vi "校准数据写入配置文件.vi"(8 "error in (no error)":errorcluster) -> (0 "error out":errorcluster)   [LabVIEW 2016, in "斯坦道通用流路CODmn.lvlib"]
uses:
  <vilib>/Utility/config.llb/NI_LVConfig.lvlib
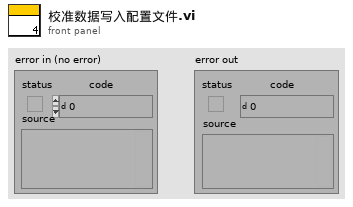
[diagram p1: front panel]
types:
  T1 = cluster{"参数":cluster{"String":string, "Value":u16}, "曲线模型":cluster{"标液浓度1":dbl, "测量吸光度1":dbl, "样品1启用":bool, "标液浓度2":dbl, "测量吸光度2":dbl, "样品2启用":bool, "标液浓度3":dbl, "测量吸光度3":dbl, "样品3启用":bool, "标液浓度4":dbl, "测量吸光度4":dbl, "样品4启用":bool, "标液浓度5":dbl, "测量吸光度5":dbl, "样品5启用":bool, "模型":enum32{"线性", "多项式"}, "精度":dbl, "XY图":cluster{"X Values":dbl[], "Y Values":dbl[]}[], "拟合公式":string, "r^2":dbl, "标样一校准时间":timestamp, "标样二校准时间":timestamp, "标样三校准时间":timestamp, "标样四校准时间":timestamp, "标样五校准时间":timestamp, "方程":cluster{"c":dbl, "x":dbl, "x^2":dbl}, "标定时间":timestamp}[]}[]
  T2 = cluster{"标液浓度1":dbl, "测量吸光度1":dbl, "样品1启用":bool, "标液浓度2":dbl, "测量吸光度2":dbl, "样品2启用":bool, "标液浓度3":dbl, "测量吸光度3":dbl, "样品3启用":bool, "标液浓度4":dbl, "测量吸光度4":dbl, "样品4启用":bool, "标液浓度5":dbl, "测量吸光度5":dbl, "样品5启用":bool, "模型":enum32{"线性", "多项式"}, "精度":dbl, "XY图":cluster{"X Values":dbl[], "Y Values":dbl[]}[], "拟合公式":string, "r^2":dbl, "标样一校准时间":timestamp, "标样二校准时间":timestamp, "标样三校准时间":timestamp, "标样四校准时间":timestamp, "标样五校准时间":timestamp, "二次方程":cluster{"c":dbl, "x":dbl, "x^2":dbl}, "标定时间":timestamp}[]
  T3 = cluster{cluster{"String":string, "Value":u16}, "总磷曲线模型":cluster{"标液浓度1":dbl, "测量吸光度1":dbl, "样品1启用":bool, "标液浓度2":dbl, "测量吸光度2":dbl, "样品2启用":bool, "标液浓度3":dbl, "测量吸光度3":dbl, "样品3启用":bool, "标液浓度4":dbl, "测量吸光度4":dbl, "样品4启用":bool, "标液浓度5":dbl, "测量吸光度5":dbl, "样品5启用":bool, "模型":enum32{"线性", "多项式"}, "精度":dbl, "XY图":cluster{"X Values":dbl[], "Y Values":dbl[]}[], "拟合公式":string, "r^2":dbl, "标样一校准时间":timestamp, "标样二校准时间":timestamp, "标样三校准时间":timestamp, "标样四校准时间":timestamp, "标样五校准时间":timestamp, "二次方程":cluster{"c":dbl, "x":dbl, "x^2":dbl}, "标定时间":timestamp}[]}
  T4 = cluster{cluster{"String":string, "Value":u16}, "总氮曲线模型":cluster{"标液浓度1":dbl, "测量吸光度1":dbl, "样品1启用":bool, "标液浓度2":dbl, "测量吸光度2":dbl, "样品2启用":bool, "标液浓度3":dbl, "测量吸光度3":dbl, "样品3启用":bool, "标液浓度4":dbl, "测量吸光度4":dbl, "样品4启用":bool, "标液浓度5":dbl, "测量吸光度5":dbl, "样品5启用":bool, "模型":enum32{"线性", "多项式"}, "精度":dbl, "XY图":cluster{"X Values":dbl[], "Y Values":dbl[]}[], "拟合公式":string, "r^2":dbl, "标样一校准时间":timestamp, "标样二校准时间":timestamp, "标样三校准时间":timestamp, "标样四校准时间":timestamp, "标样五校准时间":timestamp, "二次方程":cluster{"c":dbl, "x":dbl, "x^2":dbl}, "标定时间":timestamp}[]}
  T5 = cluster{cluster{"String":string, "Value":u16}, "氨氮曲线模型":cluster{"标液浓度1":dbl, "测量吸光度1":dbl, "样品1启用":bool, "标液浓度2":dbl, "测量吸光度2":dbl, "样品2启用":bool, "标液浓度3":dbl, "测量吸光度3":dbl, "样品3启用":bool, "标液浓度4":dbl, "测量吸光度4":dbl, "样品4启用":bool, "标液浓度5":dbl, "测量吸光度5":dbl, "样品5启用":bool, "模型":enum32{"线性", "多项式"}, "精度":dbl, "XY图":cluster{"X Values":dbl[], "Y Values":dbl[]}[], "拟合公式":string, "r^2":dbl, "标样一校准时间":timestamp, "标样二校准时间":timestamp, "标样三校准时间":timestamp, "标样四校准时间":timestamp, "标样五校准时间":timestamp, "二次方程":cluster{"c":dbl, "x":dbl, "x^2":dbl}, "标定时间":timestamp}[]}
  T6 = cluster{cluster{"String":string, "Value":u16}, "磷酸盐曲线模型":cluster{"标液浓度1":dbl, "测量吸光度1":dbl, "样品1启用":bool, "标液浓度2":dbl, "测量吸光度2":dbl, "样品2启用":bool, "标液浓度3":dbl, "测量吸光度3":dbl, "样品3启用":bool, "标液浓度4":dbl, "测量吸光度4":dbl, "样品4启用":bool, "标液浓度5":dbl, "测量吸光度5":dbl, "样品5启用":bool, "模型":enum32{"线性", "多项式"}, "精度":dbl, "XY图":cluster{"X Values":dbl[], "Y Values":dbl[]}[], "拟合公式":string, "r^2":dbl, "标样一校准时间":timestamp, "标样二校准时间":timestamp, "标样三校准时间":timestamp, "标样四校准时间":timestamp, "标样五校准时间":timestamp, "二次方程":cluster{"c":dbl, "x":dbl, "x^2":dbl}, "标定时间":timestamp}[]}
  T7 = cluster{cluster{"String":string, "Value":u16}, "硝氮曲线模型":cluster{"标液浓度1":dbl, "测量吸光度1":dbl, "样品1启用":bool, "标液浓度2":dbl, "测量吸光度2":dbl, "样品2启用":bool, "标液浓度3":dbl, "测量吸光度3":dbl, "样品3启用":bool, "标液浓度4":dbl, "测量吸光度4":dbl, "样品4启用":bool, "标液浓度5":dbl, "测量吸光度5":dbl, "样品5启用":bool, "模型":enum32{"线性", "多项式"}, "精度":dbl, "XY图":cluster{"X Values":dbl[], "Y Values":dbl[]}[], "拟合公式":string, "r^2":dbl, "标样一校准时间":timestamp, "标样二校准时间":timestamp, "标样三校准时间":timestamp, "标样四校准时间":timestamp, "标样五校准时间":timestamp, "二次方程":cluster{"c":dbl, "x":dbl, "x^2":dbl}, "标定时间":timestamp}[]}
  T8 = cluster{cluster{"String":string, "Value":u16}, "亚硝氮曲线模型":cluster{"标液浓度1":dbl, "测量吸光度1":dbl, "样品1启用":bool, "标液浓度2":dbl, "测量吸光度2":dbl, "样品2启用":bool, "标液浓度3":dbl, "测量吸光度3":dbl, "样品3启用":bool, "标液浓度4":dbl, "测量吸光度4":dbl, "样品4启用":bool, "标液浓度5":dbl, "测量吸光度5":dbl, "样品5启用":bool, "模型":enum32{"线性", "多项式"}, "精度":dbl, "XY图":cluster{"X Values":dbl[], "Y Values":dbl[]}[], "拟合公式":string, "r^2":dbl, "标样一校准时间":timestamp, "标样二校准时间":timestamp, "标样三校准时间":timestamp, "标样四校准时间":timestamp, "标样五校准时间":timestamp, "二次方程":cluster{"c":dbl, "x":dbl, "x^2":dbl}, "标定时间":timestamp}[]}
  T9 = cluster{cluster{"String":string, "Value":u16}, "硅酸盐曲线模型":cluster{"标液浓度1":dbl, "测量吸光度1":dbl, "样品1启用":bool, "标液浓度2":dbl, "测量吸光度2":dbl, "样品2启用":bool, "标液浓度3":dbl, "测量吸光度3":dbl, "样品3启用":bool, "标液浓度4":dbl, "测量吸光度4":dbl, "样品4启用":bool, "标液浓度5":dbl, "测量吸光度5":dbl, "样品5启用":bool, "模型":enum32{"线性", "多项式"}, "精度":dbl, "XY图":cluster{"X Values":dbl[], "Y Values":dbl[]}[], "拟合公式":string, "r^2":dbl, "标样一校准时间":timestamp, "标样二校准时间":timestamp, "标样三校准时间":timestamp, "标样四校准时间":timestamp, "标样五校准时间":timestamp, "二次方程":cluster{"c":dbl, "x":dbl, "x^2":dbl}, "标定时间":timestamp}[]}
  T10 = cluster{cluster{"String":string, "Value":u16}, "硫化物曲线模型":cluster{"标液浓度1":dbl, "测量吸光度1":dbl, "样品1启用":bool, "标液浓度2":dbl, "测量吸光度2":dbl, "样品2启用":bool, "标液浓度3":dbl, "测量吸光度3":dbl, "样品3启用":bool, "标液浓度4":dbl, "测量吸光度4":dbl, "样品4启用":bool, "标液浓度5":dbl, "测量吸光度5":dbl, "样品5启用":bool, "模型":enum32{"线性", "多项式"}, "精度":dbl, "XY图":cluster{"X Values":dbl[], "Y Values":dbl[]}[], "拟合公式":string, "r^2":dbl, "标样一校准时间":timestamp, "标样二校准时间":timestamp, "标样三校准时间":timestamp, "标样四校准时间":timestamp, "标样五校准时间":timestamp, "二次方程":cluster{"c":dbl, "x":dbl, "x^2":dbl}, "标定时间":timestamp}[]}
  T11 = cluster{cluster{"String":string, "Value":u16}, "CODcr曲线模型":cluster{"标液浓度1":dbl, "测量吸光度1":dbl, "样品1启用":bool, "标液浓度2":dbl, "测量吸光度2":dbl, "样品2启用":bool, "标液浓度3":dbl, "测量吸光度3":dbl, "样品3启用":bool, "标液浓度4":dbl, "测量吸光度4":dbl, "样品4启用":bool, "标液浓度5":dbl, "测量吸光度5":dbl, "样品5启用":bool, "模型":enum32{"线性", "多项式"}, "精度":dbl, "XY图":cluster{"X Values":dbl[], "Y Values":dbl[]}[], "拟合公式":string, "r^2":dbl, "标样一校准时间":timestamp, "标样二校准时间":timestamp, "标样三校准时间":timestamp, "标样四校准时间":timestamp, "标样五校准时间":timestamp, "二次方程":cluster{"c":dbl, "x":dbl, "x^2":dbl}, "标定时间":timestamp}[]}
  T12 = cluster{cluster{"String":string, "Value":u16}, "CODMn曲线模型":cluster{"标液浓度1":dbl, "测量吸光度1":dbl, "样品1启用":bool, "标液浓度2":dbl, "测量吸光度2":dbl, "样品2启用":bool, "标液浓度3":dbl, "测量吸光度3":dbl, "样品3启用":bool, "标液浓度4":dbl, "测量吸光度4":dbl, "样品4启用":bool, "标液浓度5":dbl, "测量吸光度5":dbl, "样品5启用":bool, "模型":enum32{"线性", "多项式"}, "精度":dbl, "XY图":cluster{"X Values":dbl[], "Y Values":dbl[]}[], "拟合公式":string, "r^2":dbl, "标样一校准时间":timestamp, "标样二校准时间":timestamp, "标样三校准时间":timestamp, "标样四校准时间":timestamp, "标样五校准时间":timestamp, "二次方程":cluster{"c":dbl, "x":dbl, "x^2":dbl}, "标定时间":timestamp}[]}
  T13 = cluster{cluster{"String":string, "Value":u16}, "氟化物曲线模型":cluster{"标液浓度1":dbl, "测量吸光度1":dbl, "样品1启用":bool, "标液浓度2":dbl, "测量吸光度2":dbl, "样品2启用":bool, "标液浓度3":dbl, "测量吸光度3":dbl, "样品3启用":bool, "标液浓度4":dbl, "测量吸光度4":dbl, "样品4启用":bool, "标液浓度5":dbl, "测量吸光度5":dbl, "样品5启用":bool, "模型":enum32{"线性", "多项式"}, "精度":dbl, "XY图":cluster{"X Values":dbl[], "Y Values":dbl[]}[], "拟合公式":string, "r^2":dbl, "标样一校准时间":timestamp, "标样二校准时间":timestamp, "标样三校准时间":timestamp, "标样四校准时间":timestamp, "标样五校准时间":timestamp, "二次方程":cluster{"c":dbl, "x":dbl, "x^2":dbl}, "标定时间":timestamp}[]}
  T14 = typedef "NI_LVConfig.lvlib/Config Data RefNum.ctl" = refnum<k1>
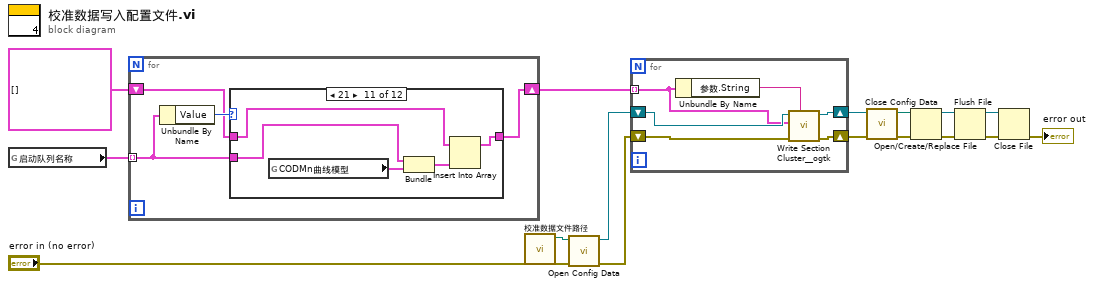
[diagram p0: block diagram]
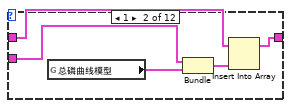
[diagram p3: hidden frame]
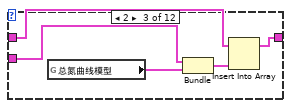
[diagram p4: hidden frame]
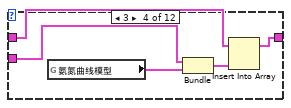
[diagram p5: hidden frame]
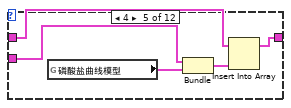
[diagram p6: hidden frame]
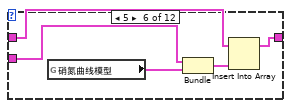
[diagram p7: hidden frame]
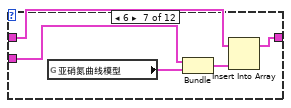
[diagram p8: hidden frame]
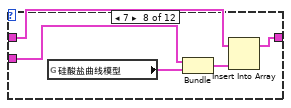
[diagram p9: hidden frame]
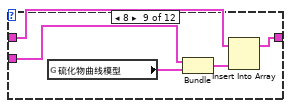
[diagram p10: hidden frame]
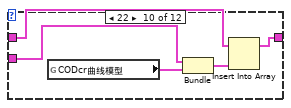
[diagram p11: hidden frame]
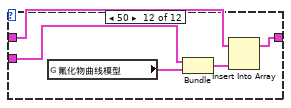
[diagram p12: hidden frame]
diagram:
  n1 = global read "model config var.vi" "启动队列名称"() -> (w12:cluster{"String":string, "Value":u16}[])
  n2 = for {
    tunnel: w12 -> [w17] mode=indexing
    shift-right: [w19] -> w11
    shift-left: T1 [] ("曲线模型") -> [w18]
    n3 = Unbundle By Name(w17) -> ("Value"=w20:u16)
    n4 = case shown="21" w20 {
      tunnel: [w21 w25 w30 w35 w40 w45 w50 w55 w60 w65 w70 w75] -> w19
      tunnel: w18 -> [w21 w26 w31 w36 w41 w46 w51 w56 w61 w66 w71 w76]
      tunnel: w17 -> [_ w23 w28 w33 w38 w43 w48 w53 w58 w63 w68 w73]
      frame 0, Default {
      }
      frame 1 {
        n5 = global read "校准数据全局变量.vi" "总磷曲线模型"() -> (w24:T2)
        n6 = Bundle(w23, "总磷曲线模型"=w24) -> (w22:T3)  [unwired: 1 in]
        n7 = Insert Into Array(array=w26, new element=w22) -> (w25:T1)  [unwired: 1 in]
      }
      frame 2 {
        n8 = global read "校准数据全局变量.vi" "总氮曲线模型"() -> (w29:T2)
        n9 = Bundle(w28, "总氮曲线模型"=w29) -> (w27:T4)  [unwired: 1 in]
        n10 = Insert Into Array(array=w31, new element=w27) -> (w30:T1)  [unwired: 1 in]
      }
      frame 3 {
        n11 = global read "校准数据全局变量.vi" "氨氮曲线模型"() -> (w34:T2)
        n12 = Bundle(w33, "氨氮曲线模型"=w34) -> (w32:T5)  [unwired: 1 in]
        n13 = Insert Into Array(array=w36, new element=w32) -> (w35:T1)  [unwired: 1 in]
      }
      frame 4 {
        n14 = global read "校准数据全局变量.vi" "磷酸盐曲线模型"() -> (w39:T2)
        n15 = Bundle(w38, "磷酸盐曲线模型"=w39) -> (w37:T6)  [unwired: 1 in]
        n16 = Insert Into Array(array=w41, new element=w37) -> (w40:T1)  [unwired: 1 in]
      }
      frame 5 {
        n17 = global read "校准数据全局变量.vi" "硝氮曲线模型"() -> (w44:T2)
        n18 = Bundle(w43, "硝氮曲线模型"=w44) -> (w42:T7)  [unwired: 1 in]
        n19 = Insert Into Array(array=w46, new element=w42) -> (w45:T1)  [unwired: 1 in]
      }
      frame 6 {
        n20 = global read "校准数据全局变量.vi" "亚硝氮曲线模型"() -> (w49:T2)
        n21 = Bundle(w48, "亚硝氮曲线模型"=w49) -> (w47:T8)  [unwired: 1 in]
        n22 = Insert Into Array(array=w51, new element=w47) -> (w50:T1)  [unwired: 1 in]
      }
      frame 7 {
        n23 = global read "校准数据全局变量.vi" "硅酸盐曲线模型"() -> (w54:T2)
        n24 = Bundle(w53, "硅酸盐曲线模型"=w54) -> (w52:T9)  [unwired: 1 in]
        n25 = Insert Into Array(array=w56, new element=w52) -> (w55:T1)  [unwired: 1 in]
      }
      frame 8 {
        n26 = global read "校准数据全局变量.vi" "硫化物曲线模型"() -> (w59:T2)
        n27 = Bundle(w58, "硫化物曲线模型"=w59) -> (w57:T10)  [unwired: 1 in]
        n28 = Insert Into Array(array=w61, new element=w57) -> (w60:T1)  [unwired: 1 in]
      }
      frame 22 {
        n29 = global read "校准数据全局变量.vi" "CODcr曲线模型"() -> (w64:T2)
        n30 = Bundle(w63, "CODcr曲线模型"=w64) -> (w62:T11)  [unwired: 1 in]
        n31 = Insert Into Array(array=w66, new element=w62) -> (w65:T1)  [unwired: 1 in]
      }
      frame 21 {
        n32 = global read "校准数据全局变量.vi" "CODMn曲线模型"() -> (w69:T2)
        n33 = Bundle(w68, "CODMn曲线模型"=w69) -> (w67:T12)  [unwired: 1 in]
        n34 = Insert Into Array(array=w71, new element=w67) -> (w70:T1)  [unwired: 1 in]
      }
      frame 50 {
        n35 = global read "校准数据全局变量.vi" "氟化物曲线模型"() -> (w74:T2)
        n36 = Bundle(w73, "氟化物曲线模型"=w74) -> (w72:T13)  [unwired: 1 in]
        n37 = Insert Into Array(array=w76, new element=w72) -> (w75:T1)  [unwired: 1 in]
      }
    }
  }
  n38 = call "校准数据文件路径.vi"() -> ("appended path"=w16:path)  [unwired: 11 in]
  n39 = call <vilib>:"Open Config Data.vi"("error in (no error)"="error in (no error)", "configuration file path"=w16) -> ("error out"=w15:errorcluster, "refnum"=w10:T14)  [unwired: 7 in, 1 out]
  n40 = for {
    shift-right: [w80] -> w9
    shift-left: w10 -> [w82]
    shift-right: [w79] -> w14
    shift-left: w15 -> [w81]
    tunnel: w11 -> [w78] mode=indexing
    n41 = Unbundle By Name(w78) -> ("参数.String"=w77:string)
    n42 = call <userlib>:"Write Section Cluster__ogtk.vi"("section (optional)"=w77, "error in (no error)"=w81, "Section Formatted Cluster"=w78, "refnum"=w82) -> ("error out"=w79:errorcluster, "dup refnum"=w80:T14)  [unwired: 6 in]
  }
  n43 = call <vilib>:"Close Config Data.vi"("error in (no error)"=w14, "refnum"=w9) -> ("error out"=w3:errorcluster, "file path"=w4:path)  [unwired: 8 in]
  n44 = Open/Create/Replace File(file path (use dialog)=w4, error in=w3) -> (refnum out=w7:refnum<file>, error out=w8:errorcluster)  [unwired: 4 in, 1 out]
  n45 = Flush File(refnum=w7, error in=w8) -> (refnum out=w6:refnum<file>, error out=w5:errorcluster)
  n46 = Close File(refnum=w6, error in=w5) -> (error out=→"error out":errorcluster)  [unwired: 1 out]
